vi "Stage 2.2 myDAQ - Filtering the signal.vi"() -> ()   [LabVIEW 2020]
panel:
  out "Filtered":waveform(dbl)(graph)
  in  "Samples s":i32=5
  out "error out":errorcluster
  out "Raw":waveform(dbl)(graph)
  in  "Stop":bool
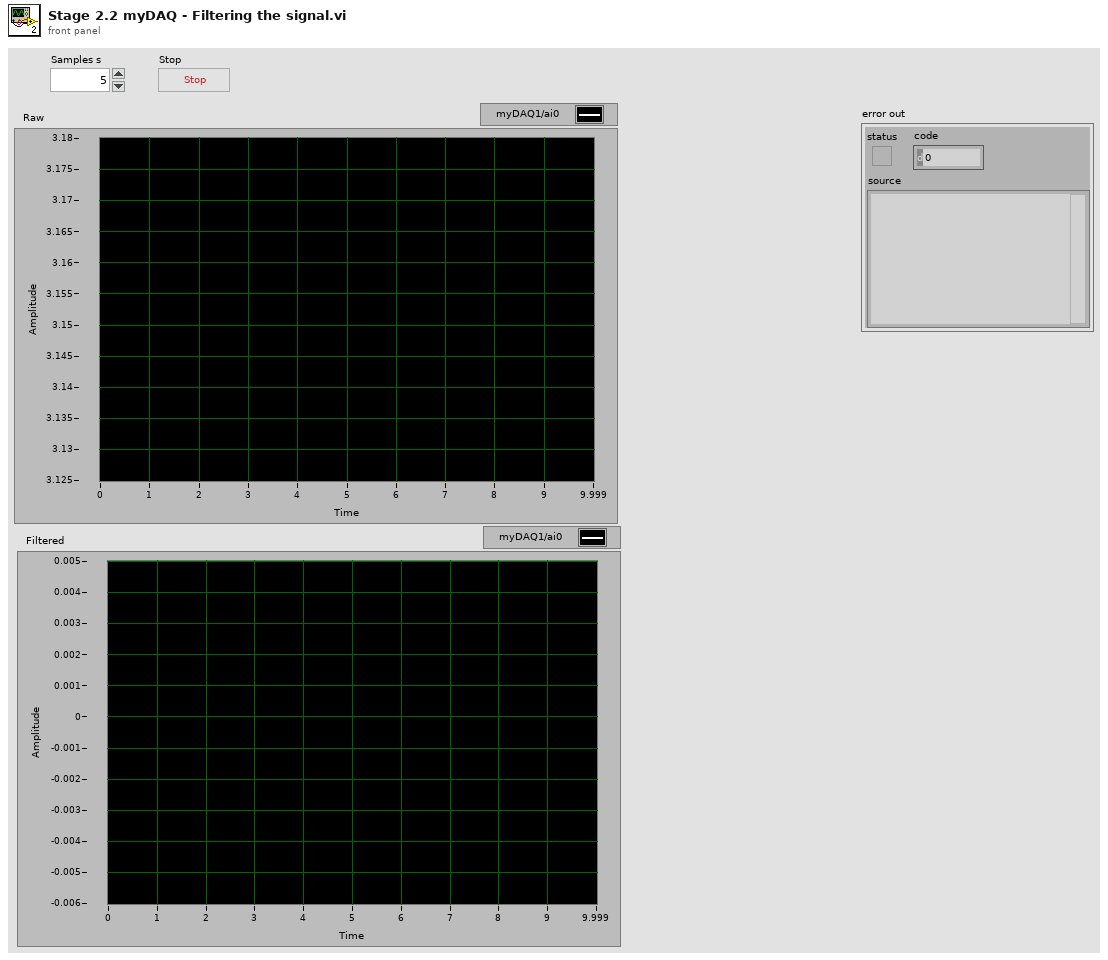
[diagram p1: front panel]
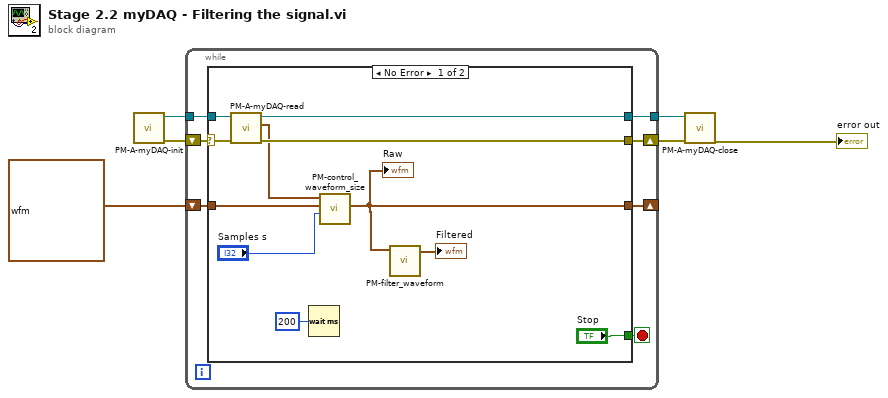
[diagram p0: block diagram]
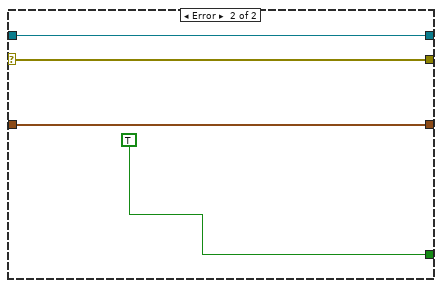
[diagram p2: hidden frame]
diagram:
  n1 = call "PM-A-myDAQ-init.vi"() -> ("error out"=w5:errorcluster, "Refnum out"=w4:refnum<k21>)  [unwired: 10 in]
  n2 = while {
    tunnel: w4 -> [w13]
    tunnel: [w11] -> w3
    shift-right: [w10] -> w2
    shift-left: w5 -> [w12]
    shift-right: [w7] -> _
    shift-left: waveform(dbl) {"t0"=timestamp(0 s since 1904-01-01), "dt"=0.0, "Y"=[]} ("data") -> [w8]
    stop <- w9 stop-if-true
    n3 = case shown="No Error" w12 {
      selector: w12 -> [w23 w27]
      tunnel: w13 -> [w24 w26]
      tunnel: [w21 w26] -> w11
      tunnel: [w20 w27] -> w10
      tunnel: ["Stop" TRUE ("Stop")] -> w9
      tunnel: w8 -> [w17 w25]
      tunnel: [w15 w25] -> w7
      frame No Error {
        n4 = call "PM-A-myDAQ-read.vi"("error in (no error)"=w23, "Refnum in"=w24) -> ("error out"=w20:errorcluster, "data"=w16:waveform(dbl), "Refnum out"=w21:refnum<k21>)  [unwired: 7 in]
        n5 = Wait (ms)(milliseconds to wait=u32 200) -> ()  [unwired: 1 out]
        n6 = call "PM-control_waveform_size.vi"("Samples s"="Samples s", "old waveform"=w17, "New waveform"=w16) -> ("waveform"=w15:waveform(dbl))  [unwired: 8 in]
        "Raw" <- w15
        n7 = call "PM-filter_waveform.vi"("waveform in"=w15) -> ("waveform out"=→"Filtered":waveform(dbl))  [unwired: 9 in, 1 out]
      }
      frame Error {
      }
    }
  }
  n8 = call "PM-A-myDAQ-close.vi"("error in (no error)"=w2, "Refnum in"=w3) -> ("error out"=→"error out":errorcluster)  [unwired: 9 in]
